vi "SubVI.vi"() -> ()   [LabVIEW 2018]
panel:
  in  "Thermoelectric Voltage":dbl
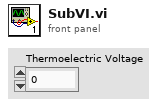
[diagram p1: front panel]
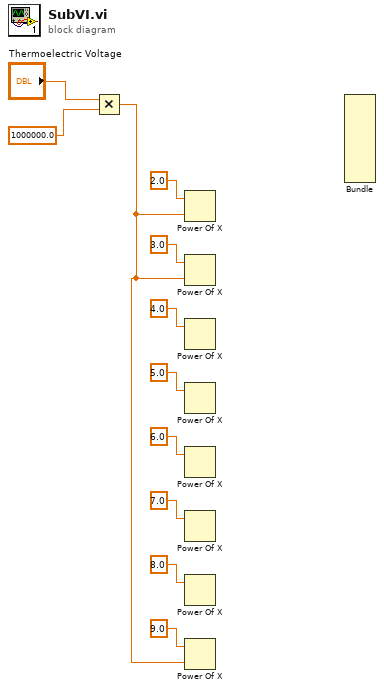
[diagram p0: block diagram]
diagram:
  n1 = Multiply(x="Thermoelectric Voltage", y=1000000.0) -> (x*y=w1:dbl)
  n2 = Power Of X(1:w1, 2:2.0 ("y")) -> ()  [unwired: 1 out]
  n3 = Power Of X(1:w1, 2:3.0 ("y")) -> ()  [unwired: 1 out]
  n4 = Power Of X(2:4.0 ("y")) -> (1:w11:dbl)  [unwired: 1 out]
  n5 = Power Of X(2:5.0 ("y")) -> (1:w9:dbl)  [unwired: 1 out]
  n6 = Power Of X(2:6.0 ("y")) -> (1:w7:dbl)  [unwired: 1 out]
  n7 = Power Of X(2:7.0 ("y")) -> (1:w5:dbl)  [unwired: 1 out]
  n8 = Power Of X(2:8.0 ("y")) -> (1:w3:dbl)  [unwired: 1 out]
  n9 = Power Of X(1:w1, 2:9.0 ("y")) -> ()  [unwired: 1 out]
  n10 = Bundle() -> ()  [unwired: 12 in, 1 out]
